vi "1 Angle to Rotational Velocity.vi"() -> ()   [LabVIEW 2011]
doc: "uses the low-pass differentiator to estimate velocity from a series of robot locations.\nTODO: does not deal with switches between UTM zones."
uses:
  2 Typedefs/heading.ctl
  2 Typedefs/rate of turn.ctl
panel:
  out "Robot\nRate of Turn":T1 format="%05.1f"
  in  "Robot\nHeading":T2 format="%05.1f"
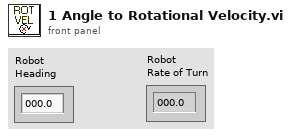
[diagram p1: front panel]
types:
  T1 = typedef "rate of turn.ctl" = dbl
  T2 = typedef "heading.ctl" = dbl
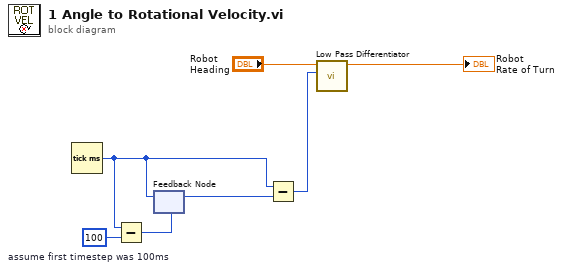
[diagram p0: block diagram]
diagram:
  w6 = u32 100  # assume first timestep was 100ms
  n1 = Tick Count (ms)() -> (millisecond timer value=w5:u32)
  n2 = Subtract(x=w5, y=w6) -> (x-y=w4:u32)
  n3 = feedback #1(w4) -> (w3:u32)
  n4 = feedback-in #1(w5) -> ()
  n5 = Subtract(x=w5, y=w3) -> (x-y=w7:u32)
  n6 = call "Low Pass Differentiator.vi"("dt"=w7, "X"="Robot\nHeading") -> ("dX, smoothed"=→"Robot\nRate of Turn":dbl)  [unwired: 9 in]
